vi "Read Write.vi"(8 "error in (no error)":errorcluster, 10 "write buffer":string, 11 "VISA Refnum in":refnum<visa-resource-name>) -> (0 "error out":errorcluster, 2 "read buffer":string, 3 "VISA Refnum out":refnum<visa-resource-name>)   [LabVIEW 2019, in "AH2500A.lvclass"]
uses:
  AH2500A.lvclass
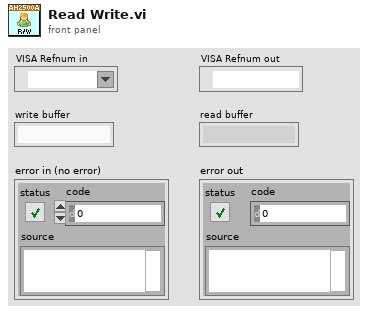
[diagram p1: front panel]
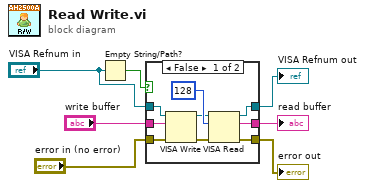
[diagram p0: block diagram]
diagram:
  n1 = Empty String/Path?(string/path="VISA Refnum in") -> (empty?=w1:bool)
  n2 = case shown="False" w1 {
    tunnel: [w16 w17] -> w7
    tunnel: [w15 w18] -> w6
    tunnel: [w14 w19] -> w5
    tunnel: "write buffer" -> [w13 w17]
    tunnel: "error in (no error)" -> [w12 w18]
    tunnel: "VISA Refnum in" -> [w8 w19]
    frame False {
      n3 = VISA Write(VISA resource name=w8, write buffer=w13, error in (no error)=w12) -> (VISA resource name out=w9:refnum<visa-resource-name>, error out=w10:errorcluster)  [unwired: 1 out]
      n4 = VISA Read(VISA resource name=w9, byte count=u32 128, error in (no error)=w10) -> (VISA resource name out=w14:refnum<visa-resource-name>, read buffer=w16:string, error out=w15:errorcluster)  [unwired: 1 out]
    }
    frame True {
    }
  }
  "read buffer" <- w7
  "error out" <- w6
  "VISA Refnum out" <- w5
